vi "GetAttributeViBoolean.vi"(8 "error in (no error)":errorcluster {"code" format="%.0x"}, 9 "AttributeID":u32(ring)=1150070 items=["DIGITIZER_MEMORY_MEASUREMENT_DATA_AUTO_SAVE_ENABLED"=1150070, "DISPLAY_ENABLED"=1150016, "FORMAT_ALARM_ENABLED"=1150023, "FORMAT_CHANNEL_ENABLED"=1150024, "FORMAT_TIME_ENABLED"=1150025, "FORMAT_UNITS_ENABLED"=1150027, "ROUTE_MONITOR_ENABLED"=1150012, "SIMULATE"=1050005, "SYSTEM_AUTOCALIBRATION_GET_ALL_MODULE_STATE"=1150051, "SYSTEM_DMM_ENABLED"=1150018, "SYSTEM_DMM_INSTALLED"=1150019, "SYSTEM_INSTRUMENT_STATE_POWER_ON_RECALL_ENABLED"=1150033, "SYSTEM_LXI_IDENTIFY_ENABLED"=1150032, "SYSTEM_TRACING_ENABLED"=1150041, "USB_MEMORY_LOGGING_ENABLED"=1150034, "USB_MEMORY_MEASUREMENT_DATA_AUTO_SAVE_ENABLED"=1150057, "USB_MEMORY_RECALL_AUTO_ENABLED"=1150052, "USB_MEMORY_ROW_LIMIT_ENABLED"=1150036], 11 "instrument handle":refnum<k15>) -> (0 "error out":errorcluster {"code" format="%.0x"}, 2 "AttributeValue":bool, 3 "instrument handle out":refnum<k15>)   [LabVIEW 2020, in "Keysight DAQ970.lvlib"]
doc: "Gets a Boolean attribute from the instrument driver.\nThe following Attributes are supported:\n\nDIGITIZER_MEMORY_MEASUREMENT_DATA_AUTO_SAVE_ENABLED\n\nDISPLAY_ENABLED\n\nFORMAT_ALARM_ENABLED\n\nFORMAT_CHANNEL_ENABLED\n\nFORMAT_TIME_ENABLED\n\nFORMAT_UNITS_ENABLED\n\nROUTE_MONITOR_ENABLED\n\nSIMULATE\n\nSYSTEM_AUTOCALIBRATION_GET_ALL_MODULE_STATE\n\nSYSTEM_DMM_ENABLED\n\nSYSTEM_DMM_INSTALLED\n\nSYSTEM_INSTRUMENT_STATE_POWER_ON_RECALL_ENABLED\n\nSYSTEM_LXI_IDENTIFY_ENABLED\n\nSYSTEM_TRACING_ENABLED\n\nUSB_MEMORY_LOGGING_ENABLED\n\nUSB_MEMORY_MEASUREMENT_DATA_AUTO_SAVE_ENABLED\n\nUSB_MEMORY_RECALL_AUTO_ENABLED\n\nUSB_MEMORY_ROW_LIMIT_ENABLED"
uses:
  Keysight DAQ970.lvlib
  KtDAQ970.dll
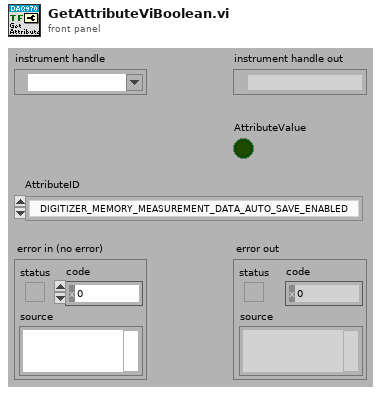
[diagram p1: front panel]
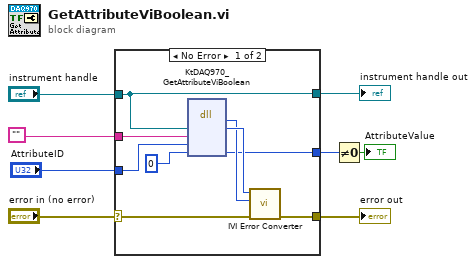
[diagram p0: block diagram]
diagram:
  n1 = case shown="No Error" "error in (no error)" {
    selector: "error in (no error)" -> [w15 w19]
    tunnel: [w14 w19] -> w8
    tunnel: "instrument handle" -> [w9 w18]
    tunnel: "" -> [w13 _]
    tunnel: "AttributeID" -> [w12 _]
    tunnel: [w10 _] -> w4
    tunnel: [w9 w18] -> w3
    frame No Error {
      n2 = dll-call lib="KtDAQ970**.dll" fn="KtDAQ970_GetAttributeViBoolean"("Vi"=w9, "RepCapIdentifier"=w13, "AttributeID"=w12, "AttributeValue"=i16 0) -> ("return type"=w16:i32, "Vi"=w17:u32, "AttributeValue"=w10:i16)  [unwired: 5 in, 2 out]
      n3 = call "IVI Error Converter.vi"("error in (no error)"=w15, "IVI error code (0)"=w16, "instrument handle"=w17) -> ("error out"=w14:errorcluster)  [unwired: 7 in, 1 out]
    }
    frame Error {
    }
  }
  "error out" <- w8
  "instrument handle out" <- w3
  n4 = Not Equal To 0?(x=w4) -> (x != 0?=→"AttributeValue":bool)
